vi "Check Bounds.vi"(5 "source vi name":string, 7 "buffer size":u64 format="%d bytes", 8 "error in (no error)":errorcluster, 9 "offset (0)":u64 format="%d bytes", 10 "size to move":u64 format="%d bytes", 11 "Pointer in":refnum<class "Pointer.lvclass">) -> (0 "error out":errorcluster, 1 "offset":u64 format="%d bytes", 2 "size to move":u64 format="%d bytes", 3 "Pointer out":refnum<class "Pointer.lvclass">)   [LabVIEW 2027, in "Memory Manager.lvlib" / "Pointer.lvclass"]
uses:
  Pointer.lvclass
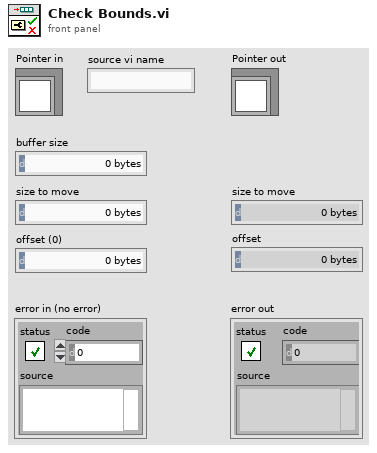
[diagram p1: front panel]
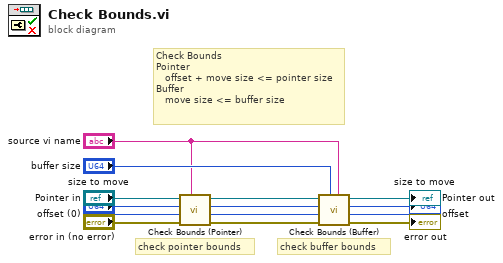
[diagram p0: block diagram]
diagram:
  # "check buffer bounds"
  # "check pointer bounds"
  # "Check Bounds\nPointer\n   offset + move size <= pointer size\nBuffer\n   move size <= buffer size"
  n1 = call "Check Bounds (Pointer).vi"("source vi name"="source vi name", "error in (no error)"="error in (no error)", "offset (0)"="offset (0)", "size"="size to move", "Pointer in"="Pointer in") -> ("error out"=w9:errorcluster, "offset out"=w7:u64, "size"=w8:u64, "Pointer out"=w10:refnum<class "Pointer.lvclass">)  [unwired: 3 in]
  n2 = call "Check Bounds (Buffer).vi"("source vi name"="source vi name", "buffer size"="buffer size", "error in (no error)"=w9, "offset (0)"=w7, "size to move"=w8, "Pointer in"=w10) -> ("error out"=→"error out":errorcluster, "offset"=→"offset":u64, "size to move"=→"size to move":u64, "Pointer out"=→"Pointer out":refnum<class "Pointer.lvclass">)  [unwired: 2 in]
